vi "RT Read From Serial.vi"(7 "Message Queue":refnum<queue>, 8 "error in (no error)":errorcluster, 9 "FPGA VI Reference":refnum<k20>, 10 "timeout (ms)":u32=2000, 11 "port name in":refnum<visa-resource-name>) -> (0 "error out":errorcluster, 1 "expect response?":bool, 2 "reading successfully done?":bool, 3 "port name out":refnum<visa-resource-name>, 5 "request received":string)   [LabVIEW 2018]
uses:
  Message Queue/Message Cluster.ctl
  <vilib>/NI_Real-Time Target Support.lvlib
  Message Queue/Message Queue.lvlib
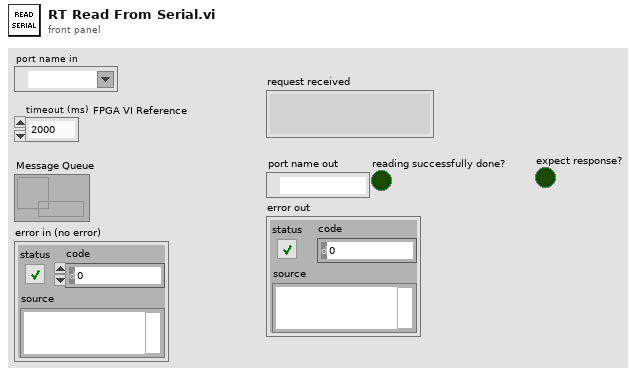
[diagram p1: front panel]
types:
  T1 = cluster{"2: expecting response?":bool, "expected max length":u32}
  T2 = cluster{"1: do writing?":bool, "write buffer":string}
  T3 = cluster{"0. connect/reconnect?":bool, "last: disconnect?":bool, "slow serial port init delay":u32}
  T4 = cluster{"read timeout?":bool, "return count":u32, "read buffer":string}
  T5 = typedef "FPGA parameter cluster.ctl" = cluster{"Output settings":cluster{"Relay Switch Matrix":u32, "Set output":sgl[], "set output?":bool, "set relay matrix?":bool}, "PID settings":cluster{"PID input channel":enum16{"Output Channel 0", "Output Channel 1", "Output Channel 2", "Output Channel 3", "PID Disabled"}, "PID output channel":enum16{"Output Channel 0", "Output Channel 1", "Output Channel 2", "Output Channel 3", "PID Disabled"}, "PID gains":cluster{"proportional gain":sgl, "integral gain":sgl, "derivative gain":sgl, "filter coefficient":sgl}, "PID output ranges":cluster{"output high (Inf)":sgl, "output low (-Inf)":sgl}, "Setpoint for PID input chn":sgl, "config PID gain?":bool, "reset PID?":bool, "config PID range?":bool, "config PID input?":bool, "config PID output?":bool, "config PID setpoint?":bool}, "NI9219 Settings":cluster{"9219 Conversion Time":enum8{"High Speed", "Best 60 Hz Rejection", "Best 50 Hz Rejection", "High Resolution"}, "Input voltage range":T6[], "config 9219 conversion time?":bool, "config 9219 input range?":bool}, "REQUEST_ID":u64, "requests":cluster{"request_data":bool, "request_system_status":bool, "request_error_log":bool}}
  T6 = typedef "NI9219VoltageRange.ctl" = u8
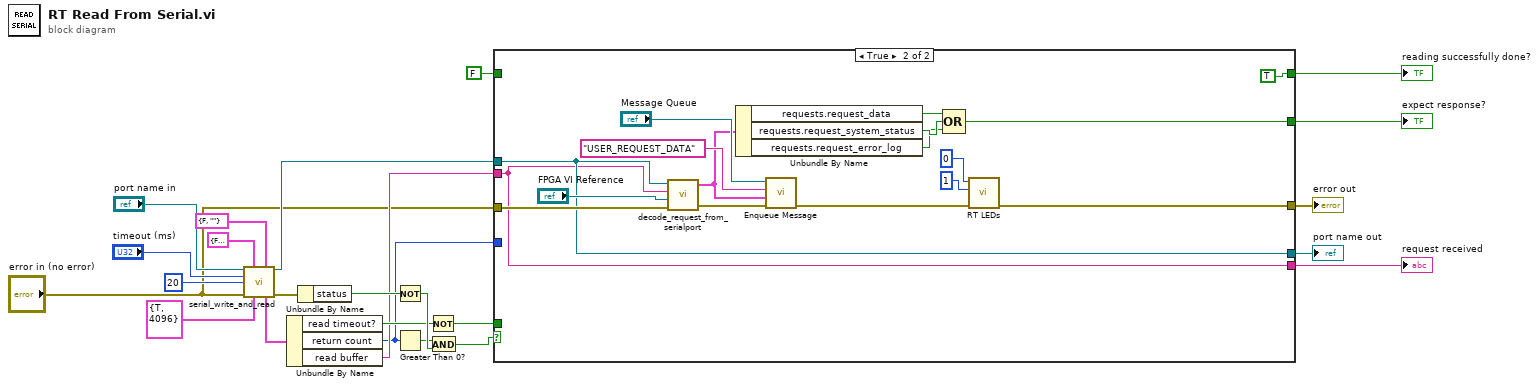
[diagram p0: block diagram]
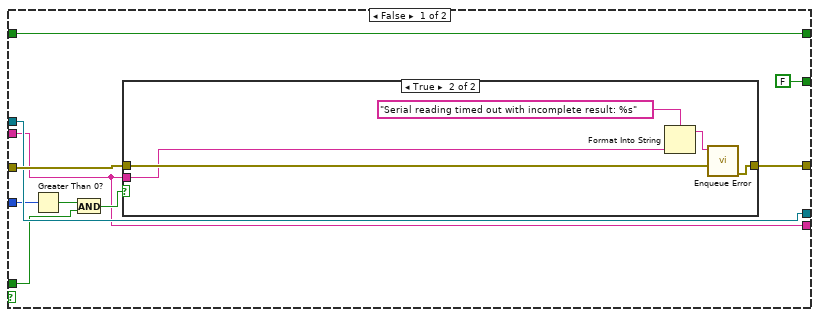
[diagram p2: hidden frame]
diagram:
  n1 = call "serial_write_and_read.vi"("port name in"="port name in", "0 and last: Connection/Reconnection setting"=T3 {"0. connect/reconnect?"=FALSE, "last: disconnect?"=FALSE, "slow serial port init delay"=0}, "1. writing setting input"=T2 {"1: do writing?"=FALSE, "write buffer"=""}, "total operation timeout (ms)"="timeout (ms)", "waiting interval between reading scans (ms)"=u32 20, "error in"="error in (no error)", "2. reading settings input"=T1 {"2: expecting response?"=TRUE, "expected max length"=4096}) -> ("port name out"=w15:refnum<visa-resource-name>, "reading output"=w9:T4, "error out"=w14:errorcluster)  [unwired: 6 in]
  n2 = Unbundle By Name(w9) -> ("read timeout?"=w8:bool, "return count"=w5:u32, "read buffer"=w6:string)
  n3 = Unbundle By Name(w14) -> ("status"=w18:bool)
  n4 = Not(x=w18) -> (.not. x?=w17:bool)
  n5 = Greater Than 0?(x=w5) -> (x > 0?=w13:bool)
  n6 = Not(x=w8) -> (.not. x?=w7:bool)
  n7 = And(x=w13, y=w17) -> (x .and. y?=w16:bool)
  n8 = case shown="True" w16 {
    tunnel: w15 -> [w32 w48]
    tunnel: "error in (no error)" -> [w34 w56]
    tunnel: [w33 w49] -> w23
    tunnel: [w32 w48] -> w24
    tunnel: FALSE -> [w31 _]
    tunnel: [w31 TRUE] -> w21
    tunnel: w6 -> [w27 w41]
    tunnel: [FALSE w42] -> w19
    tunnel: [w27 w41] -> w20
    tunnel: w7 -> [w25 _]
    tunnel: w5 -> [w26 _]
    frame False {
      n9 = Greater Than 0?(x=w26) -> (x > 0?=w29:bool)
      n10 = And(x=w29, y=w25) -> (x .and. y?=w28:bool)
      n11 = case shown="True" w28 {
        tunnel: w34 -> [w35 w40]
        tunnel: [w35 w37] -> w33
        tunnel: w27 -> [_ w36]
        frame False {
        }
        frame True {
          n12 = Format Into String(format string="Serial reading timed out with incomplete result: %s" ("Block information (which loop the error happens)"), w36) -> (resulting string=w38:string)  [unwired: 2 in, 1 out]
          n13 = call "Enqueue Error.vi"("error to process"=w40, "Block information (which loop the error happens)"=w38) -> ("error out"=w37:errorcluster)  [unwired: 9 in]
        }
      }
    }
    frame True {
      n14 = call "decode_request_from_serialport.vi"("error in"=w56, "FPGA VI Reference"="FPGA VI Reference", "request string"=w41, "port name in"=w48) -> ("error out"=w51:errorcluster, "FPGA settings"=w46:T5)  [unwired: 1 in]
      n15 = Unbundle By Name(w46) -> ("requests.request_data"=w45:bool, "requests.request_system_status"=w44:bool, "requests.request_error_log"=w43:bool)
      n16 = call "Enqueue Message.vi"("error in (no error)"=w51, "Message Data"=w46, "Message"="USER_REQUEST_DATA", "Message Queue"="Message Queue") -> ("error out"=w50:errorcluster)  [unwired: 6 in, 1 out]
      n17 = Compound Arithmetic op=OR(w45, w44, w43) -> (w42:bool)
      n18 = call <vilib>:"RT LEDs.vi"("error in (no error)"=w50, "State"=1, "LED Num"=0) -> ("error out"=w49:errorcluster)  [unwired: 3 in, 1 out]
    }
  }
  "port name out" <- w24
  "error out" <- w23
  "reading successfully done?" <- w21
  "request received" <- w20
  "expect response?" <- w19
